vi "generateInternalProcessCommand.vi"(8 "error in (no error)":errorcluster, 10 "ProcessCommandEvent":T1, 11 "UserEvents in":refnum<class "UserEvents.lvclass">) -> (0 "error out":errorcluster, 3 "UserEvents out":refnum<class "UserEvents.lvclass">)   [LabVIEW 2016, in "UserEvents.lvclass"]
uses:
  UserEvents.lvclass
  DataTypes/General/ProcessCommandEvent.ctl
  Commands/Command/Command.lvclass
  UserEvents.lvclass/UserEvents.ctl
  DataTypes/General/M1M3SupportGeneral.lvlib
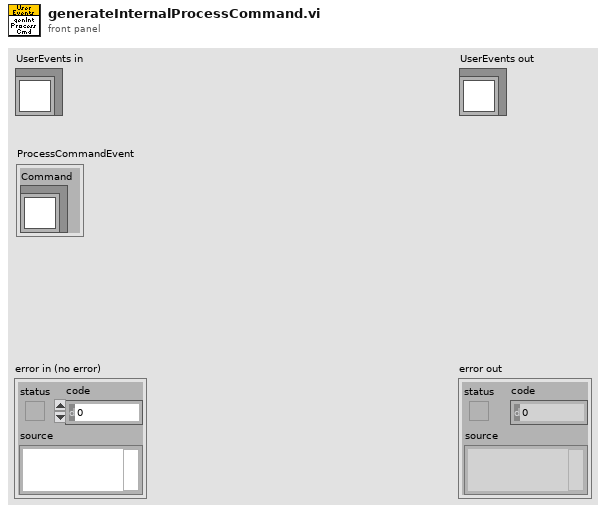
[diagram p1: front panel]
types:
  T1 = typedef "M1M3SupportGeneral.lvlib/ProcessCommandEvent.ctl" = cluster{"Command":refnum<class "Command.lvclass">}
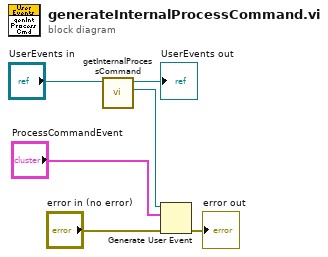
[diagram p0: block diagram]
diagram:
  n1 = call "getInternalProcessCommand.vi"("UserEvents in"="UserEvents in") -> ("InternalProcessCommand"=w5:refnum<user-event>, "UserEvents out"=→"UserEvents out":refnum<class "UserEvents.lvclass">)  [unwired: 9 in]
  n2 = Generate User Event(user event=w5, event data cluster="ProcessCommandEvent", error in="error in (no error)") -> (error out=→"error out":errorcluster)  [unwired: 1 in, 1 out]
